vi "Begin.vi"(8 "error in":errorcluster) -> (0 "error out":errorcluster)   [LabVIEW 2023]
doc: "Called before other user functions, this VI can be used to open I/O refnums, load in file data, and do general program initialization. Notice that the <B>error out</B> terminal is simply used for data flow. Wiring it to other structures or subVIs ensures that this VI runs first."
uses:
  <vilib>/Rock Robotics/WPI/DriverStation/WPI_DriverStationRobotMode2.ctl
  <vilib>/Rock Robotics/WPI/Joystick/WPI_JoystickDeviceEnum.ctl
  Swerve/Implementation/Swerve Setpoints2.ctl
  Swerve/Implementation/Swerve Operations.ctl
  <vilib>/Rock Robotics/SystemInterfaces/DIO/FPGA_DIOChannel.ctl
  <vilib>/Rock Robotics/WPI/SafetyOutput/WPI_SafetyOutputConfigMenu.ctl
  <vilib>/Rock Robotics/WPI/ThirdParty/REV Robotics/REVLib/Typedef/Spark MAX Sensor Type.ctl
  <vilib>/Rock Robotics/WPI/ThirdParty/Phoenix-LabVIEW/Motor Controller/Controls/CTRE_Phoenix_MotorControl_NeutralMode.ctl
  <vilib>/Rock Robotics/WPI/ThirdParty/REV Robotics/REVLib/Typedef/Spark MAX Idle Mode.ctl
  Robot Global Data.vi
  <vilib>/Rock Robotics/Network Tables/NT Write String Array.vi
  <vilib>/Rock Robotics/SystemInterfaces/DIO/FPGA_DIOPWMChannel.ctl
panel:
  in  "Swerve PID":T1={"P Gain"=1.1, "I Gain"=0.0, "D Gain"=0.0, "F Gain"=0.0, "I Zone"=0.0, "Min Output"=-1.0, "Max Output"=1.0}
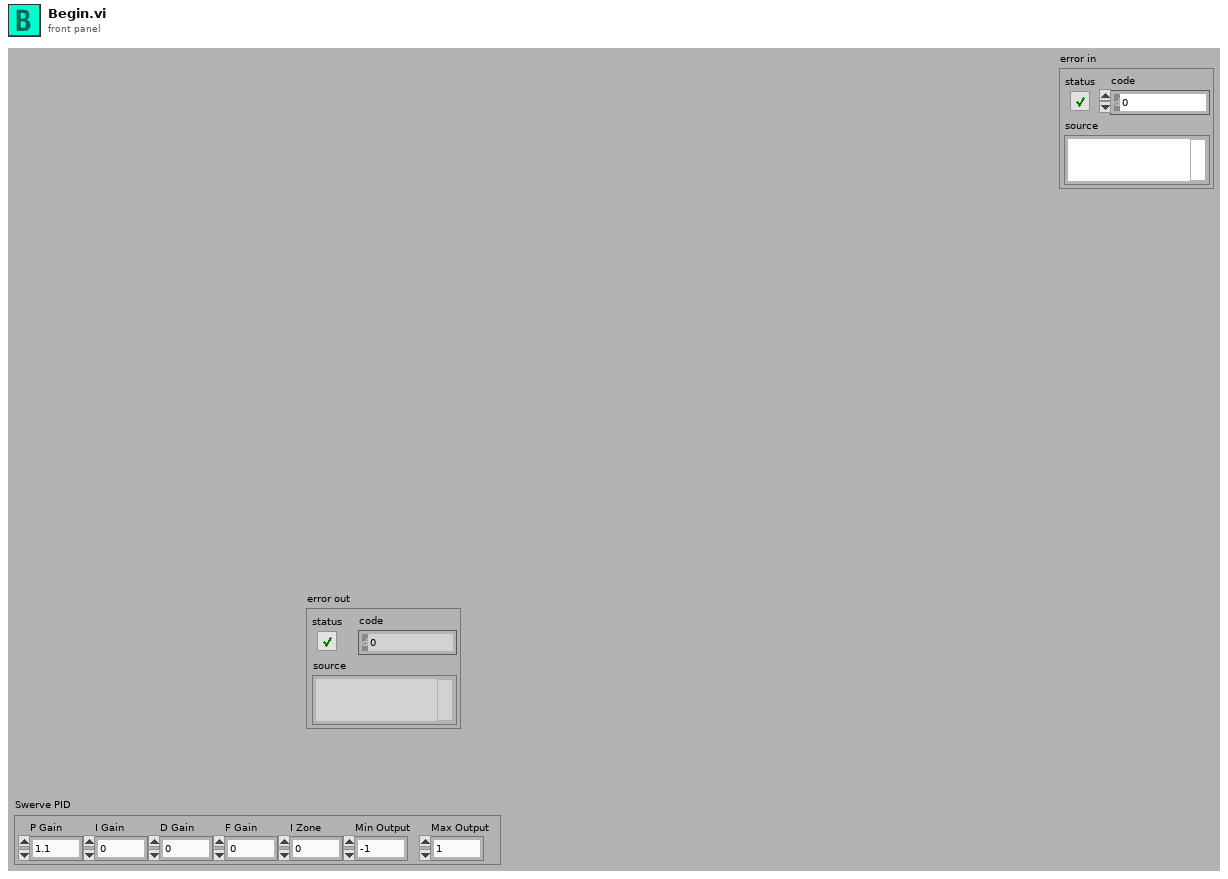
[diagram p1: front panel]
types:
  T1 = cluster{"P Gain":dbl, "I Gain":dbl, "D Gain":dbl, "F Gain":dbl, "I Zone":dbl, "Min Output":dbl, "Max Output":dbl}
  T2 = typedef "FPGA_DIOChannel.ctl" = enum8{"DIO 0", "DIO 1", "DIO 2", "DIO 3", "DIO 4", "DIO 5", "DIO 6", "DIO 7", "DIO 8", "DIO 9", "DIO MXP 0", "DIO MXP 1", "DIO MXP 2", "DIO MXP 3", "DIO MXP 4", "DIO MXP 5", "DIO MXP 6", "DIO MXP 7", "DIO MXP 8", "DIO MXP 9", "DIO MXP 10", "DIO MXP 11", "DIO MXP 12", "DIO MXP 13", "DIO MXP 14", "DIO MXP 15", "SPI Port CS1", "SPI Port CS2", "SPI Port CS3", "SPI Port MISO", "SPI Port MOSI", "Invalid"}
  T3 = typedef "Swerve Setpoints2.ctl" = cluster{"Operation":T4, "Gyro":dbl, "FWD":dbl, "STR":dbl, "X rotate":dbl, "Y rotate":dbl, "Time":dbl, "Distance":dbl, "Right Trigger":dbl, "Angle":dbl, "Start Angle":dbl, "Tag ID":dbl, "Start Positions":dbl[]}
  T4 = typedef "Swerve Operations.ctl" = enum16{"Reserve", "Read Current", "Immediate", "Stop", "Balance", "Direct  Joystick Drive", "Joystick Drive", "Drive for Distance", "Drive for Time", "Turn to Angle", "Drive to Angle(Time)", "Drive to Angle(Distance)", "Look At Cone", "Look At Cube", "Move To Tape", "Move To Tag"}
  T5 = typedef "WPI_JoystickDeviceEnum.ctl" = enum16{"USB 0", "USB 1", "USB 2", "USB 3", "USB 4", "USB 5"}
  T6 = typedef "WPI_DriverStationRobotMode2.ctl" = enum16{"Autonomous Disabled", "Autonomous Enabled", "Teleop Disabled", "Teleop Enabled", "Disconnected", "Finish", "Test Disabled", "Test Enabled", "Emergency Stopped"}
  T7 = typedef "Spark MAX Sensor Type.ctl" = enum16{"No Sensor", "Hall Sensor", "Encoder", "-Not Available-", "Analog", "Alternate Encoder", "Duty Cycle"}
  T8 = typedef "Spark MAX Idle Mode.ctl" = enum16{"Coast", "Brake"}
  T9 = typedef "WPI_SafetyOutputConfigMenu.ctl" = enum16{"Enable", "Disable"}
  T10 = typedef "WPI_MotorControlDeviceRef.ctl" = cluster{"DeviceStatus":errorcluster, "Type":T11, "PWM":cluster{"PWM Channel":T12, "DeadBand":T13}, "CAN":cluster{"Device Number":u8, "SetOutput VI Ref":variant, "GetOutput VI Ref":variant, "Enable VI Ref":variant, "Disable VI Ref":variant, "Data":variant}, "Invert":bool, "DIO PWM":cluster{"PWM \"Enable\" Channel":T12, "DIOChannel":T2, "PWM Rate":dbl}}
  T11 = typedef "WPI_MotorControlType.ctl" = enum16{"PWM", "CAN", "DIO PWM"}
  T12 = typedef "FPGA_DIOPWMChannel.ctl" = enum8{"PWM 0", "PWM 1", "PWM 2", "PWM 3", "PWM 4", "PWM 5", "PWM 6", "PWM 7", "PWM 8", "PWM 9", "PWM MXP 0", "PWM MXP 1", "PWM MXP 2", "PWM MXP 3", "PWM MXP 4", "PWM MXP 5", "PWM MXP 6", "PWM MXP 7", "PWM MXP 8", "PWM MXP 9", "Invalid"}
  T13 = typedef "WPI_PWMDeadband.ctl" = cluster{"Name":string, "maxPositivePwm":i32, "minPositivePwm":i32, "centerPwm":i32, "maxNegativePwm":i32, "minNegativePwm":i32, "angularRange":u16}
  T14 = typedef "WPI_JoystickDevRef.ctl" = cluster{"Device":T5}
  T15 = typedef "ADIS16470 Device Reference.ctl" = cluster{"DevStatus":errorcluster, "Hardware Config":T16, "Calibration Complete":refnum<notifier>, "Status Reference":refnum<data-value>, "Data Reference":refnum<data-value>, "Sychronous Process VI":T19, "Cmd FIFO":refnum<k33>, "Source":T20, "Data FIFO":refnum<k33>, "Calibration Time (ms)":u32, "Data Reference":refnum<data-value>}
  T16 = typedef "ADIS16470 Hardware Configuration.ctl" = cluster{"SPI Clock Rate (Hz)":dbl, "IMU SPI Mode (3)":T17, "IMU Reset Pin":T2, "IMU SPI Bus":T18, "IMU Data Ready Pin":T2, "Stall Config":cluster{"Pow2BytesPerRead":u8, "StallTicks":u16, "CsToSclkTicks":u8}}
  T17 = typedef "WPI_SPIMode.ctl" = enum16{"Mode 0 (Clk Idle Low,Sample on Leading)", "Mode 1 (Clk Idle Low,Sample on Trailing)", "Mode 2 (Clk Idle High,Sample on Leading)", "Mode 3 (Clk Idle High,Sample on Trailing)"}
  T18 = typedef "spi_bus.ctl" = enum16{"SPI On-Board, CS0", "SPI On-Board, CS1", "SPI On-Board, CS2", "SPI On-Board, CS3", "SPI MXP", "Invalid"}
  T19 = typedef "ADIS16470 Process.ctl" = refnum<vi>
  T20 = typedef "FPGA_CounterEncoderSourceConvertionLVSourceType.ctl" = cluster{"DevStatus":errorcluster, "AnalogTriggerMode?":bool, "DigitalMode":cluster{"DIO Channel":T21}, "AnalogTriggerMode":cluster{"AnalogTriggerIndex":T22, "OutputType":T23}}
  T21 = typedef "FPGA_DIODigitalSourceChannel.ctl" = enum8{"DIO 0", "DIO 1", "DIO 2", "DIO 3", "DIO 4", "DIO 5", "DIO 6", "DIO 7", "DIO 8", "DIO 9", "DIO MXP 0", "DIO MXP 1", "DIO MXP 2", "DIO MXP 3", "DIO MXP 4", "DIO MXP 5", "DIO MXP 6", "DIO MXP 7", "DIO MXP 8", "DIO MXP 9", "DIO MXP 10", "DIO MXP 11", "DIO MXP 12", "DIO MXP 13", "DIO MXP 14", "DIO MXP 15", "SPI Port CS1", "SPI Port CS2", "SPI Port CS3", "SPI Port MISO", "SPI Port MOSI", "Disabled"}
  T22 = typedef "FPGA_AnalogTriggerIndex.ctl" = enum8{"Trig 0", "Trig 1", "Trig 2", "Trig 3", "Trig 4", "Trig 5", "Trig 6", "Trig 7", "Invalid"}
  T23 = typedef "FPGA_AnalogTriggerOutType.ctl" = enum16{"InWindow", "TriggerState", "Rising", "Falling"}
  T24 = typedef "WPI_DigitalInputDevRef.ctl" = cluster{"DevStatus":errorcluster, "DIO Channel":T2}
  T25 = typedef "CTRE_Phoenix_MotorControl_NeutralMode.ctl" = enum8{"EEPROMSetting", "Override to Coast", "Override to Brake"}
  T26 = typedef "WPI_PWMDeviceRef.ctl" = cluster{"DeviceStatus":errorcluster, "PWM Channel":T12}
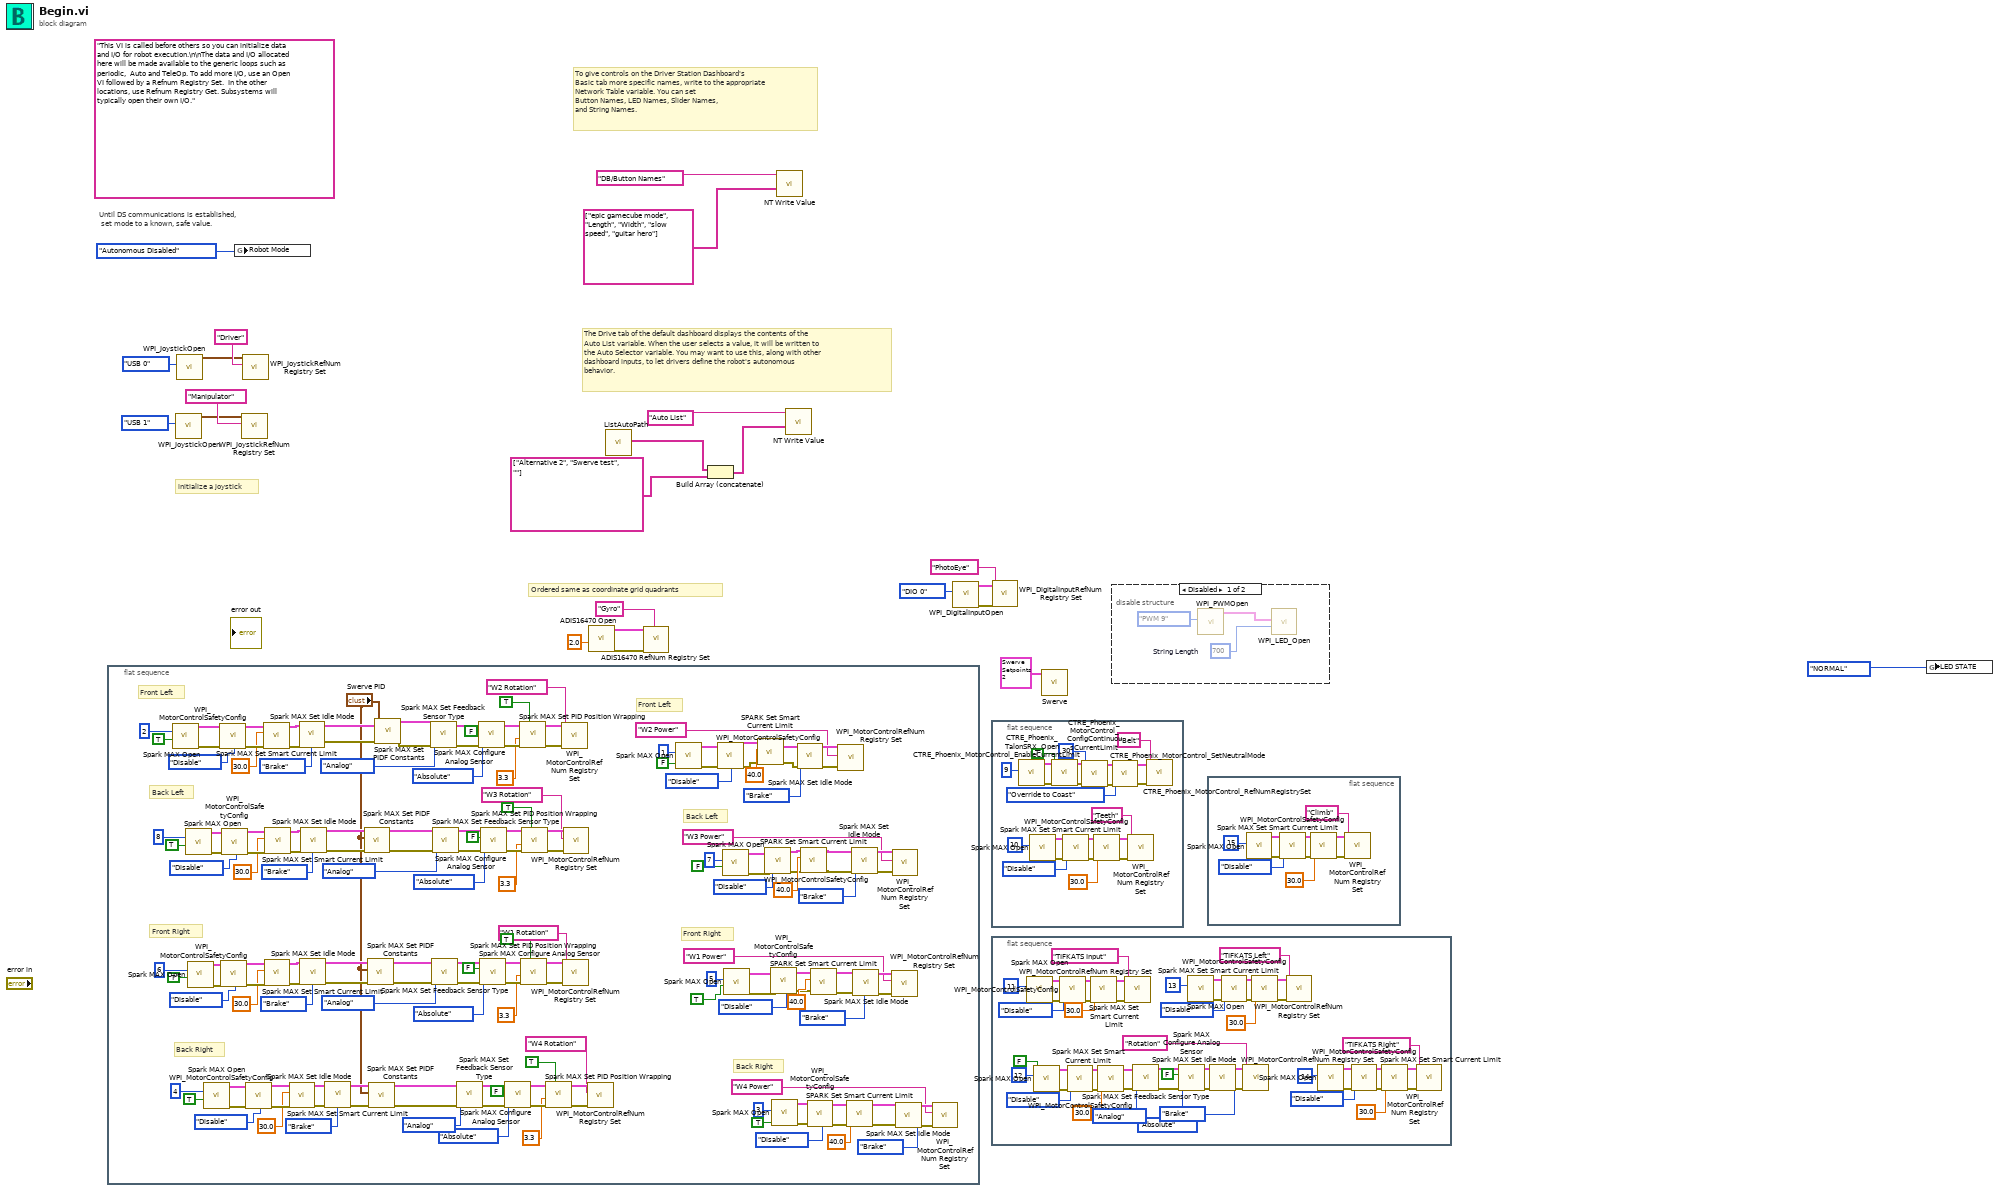
[diagram p0: block diagram]
diagram:
  (unwired) "This VI is called before others so you can initialize data and I/O for robot execution.\n\nThe data and I/O allocated here will be made available to the generic loops such as periodic,  Auto and TeleOp. To add more I/O, use an Open VI followed by a Refnum Registry Set.  In the other locations, use Refnum Registry Get. Subsystems will typically open their own I/O."
  # "Ordered same as coordinate grid quadrants"
  # "The Drive tab of the default dashboard displays the contents of the\nAuto List variable. When the user selects a value, it will be written to\nthe Auto Selector variable. You may want to use this, along with other\ndashboard inputs, to let drivers define the robot's autonomous\nbehavior."
  # "To give controls on the Driver Station Dashboard's\nBasic tab more specific names, write to the appropriate\nNetwork Table variable. You can set\nButton Names, LED Names, Slider Names,\nand String Names."
  # "initialize a joystick"
  # "Until DS communications is established,\n set mode to a known, safe value."
  n1 = flat-sequence {
    frame #0 {
      # "Back Right"
      # "Back Right"
      # "Front Right"
      # "Front Right"
      # "Back Left"
      # "Back Left"
      # "Front Left"
      # "Front Left"
      n2 = call <vilib>:"Spark MAX Open.vi"("Invert"=TRUE, "Device Number"=u8 2) -> ("error out"=w106:errorcluster, "MotorControlDeviceRef"=w107:T10)  [unwired: 8 in]
      n3 = call <vilib>:"Spark MAX Open.vi"("Invert"=TRUE, "Device Number"=u8 8) -> ("error out"=w170:errorcluster, "MotorControlDeviceRef"=w171:T10)  [unwired: 8 in]
      n4 = call <vilib>:"Spark MAX Open.vi"("Invert"=TRUE, "Device Number"=u8 6) -> ("error out"=w86:errorcluster, "MotorControlDeviceRef"=w87:T10)  [unwired: 8 in]
      n5 = call <vilib>:"Spark MAX Open.vi"("Invert"=TRUE, "Device Number"=u8 4) -> ("error out"=w66:errorcluster, "MotorControlDeviceRef"=w67:T10)  [unwired: 8 in]
      n6 = call <vilib>:"WPI_MotorControlSafetyConfig.vi"("error in (no error)"=w106, "mode"=WPI_SafetyOutputConfigMenu."Disable", "MotorControlDevRef"=w107) -> ("error out"=w124:errorcluster, "MotorControlDevRef"=w122:T10)  [unwired: 7 in]
      n7 = call <vilib>:"WPI_MotorControlSafetyConfig.vi"("error in (no error)"=w86, "mode"=WPI_SafetyOutputConfigMenu."Disable", "MotorControlDevRef"=w87) -> ("error out"=w104:errorcluster, "MotorControlDevRef"=w102:T10)  [unwired: 7 in]
      n8 = call <vilib>:"WPI_MotorControlSafetyConfig.vi"("error in (no error)"=w170, "mode"=WPI_SafetyOutputConfigMenu."Disable", "MotorControlDevRef"=w171) -> ("error out"=w178:errorcluster, "MotorControlDevRef"=w174:T10)  [unwired: 7 in]
      n9 = call <vilib>:"WPI_MotorControlSafetyConfig.vi"("error in (no error)"=w66, "mode"=WPI_SafetyOutputConfigMenu."Disable", "MotorControlDevRef"=w67) -> ("error out"=w84:errorcluster, "MotorControlDevRef"=w82:T10)  [unwired: 7 in]
      n10 = call <vilib>:"Spark MAX Set Smart Current Limit.vi"("error in (no error)"=w124, "Primay Current Limit (80A)"=30.0, "MotorControlDeviceRef in"=w122) -> ("error out"=w125:errorcluster, "MotorControlDeviceRef out"=w123:T10)  [unwired: 7 in]
      n11 = call <vilib>:"Spark MAX Set Smart Current Limit.vi"("error in (no error)"=w104, "Primay Current Limit (80A)"=30.0, "MotorControlDeviceRef in"=w102) -> ("error out"=w105:errorcluster, "MotorControlDeviceRef out"=w103:T10)  [unwired: 7 in]
      n12 = call <vilib>:"Spark MAX Set Smart Current Limit.vi"("error in (no error)"=w178, "Primay Current Limit (80A)"=30.0, "MotorControlDeviceRef in"=w174) -> ("error out"=w179:errorcluster, "MotorControlDeviceRef out"=w175:T10)  [unwired: 7 in]
      n13 = call <vilib>:"Spark MAX Set Smart Current Limit.vi"("error in (no error)"=w84, "Primay Current Limit (80A)"=30.0, "MotorControlDeviceRef in"=w82) -> ("error out"=w85:errorcluster, "MotorControlDeviceRef out"=w83:T10)  [unwired: 7 in]
      n14 = call <vilib>:"Spark MAX Set Idle Mode.vi"("error in (no error)"=w125, "Idle Mode"=Spark_MAX_Idle_Mode."Brake", "MotorControlDeviceRef in"=w123) -> ("error out"=w57:errorcluster, "MotorControlDeviceRef out"=w56:T10)  [unwired: 7 in]
      n15 = call <vilib>:"Spark MAX Set Idle Mode.vi"("error in (no error)"=w105, "Idle Mode"=Spark_MAX_Idle_Mode."Brake", "MotorControlDeviceRef in"=w103) -> ("error out"=w49:errorcluster, "MotorControlDeviceRef out"=w50:T10)  [unwired: 7 in]
      n16 = call <vilib>:"Spark MAX Set Idle Mode.vi"("error in (no error)"=w179, "Idle Mode"=Spark_MAX_Idle_Mode."Brake", "MotorControlDeviceRef in"=w175) -> ("error out"=w53:errorcluster, "MotorControlDeviceRef out"=w54:T10)  [unwired: 7 in]
      n17 = call <vilib>:"Spark MAX Set Idle Mode.vi"("error in (no error)"=w85, "Idle Mode"=Spark_MAX_Idle_Mode."Brake", "MotorControlDeviceRef in"=w83) -> ("error out"=w45:errorcluster, "MotorControlDeviceRef out"=w46:T10)  [unwired: 7 in]
      n18 = call <vilib>:"Spark MAX Set PIDF Constants.vi"("error in"=w53, "PID Constants"="Swerve PID", "MotorControlDeviceRef"=w54) -> ("error out"=w51:errorcluster, "MotorControlDeviceRef"=w52:T10)  [unwired: 7 in]
      n19 = call <vilib>:"Spark MAX Set PIDF Constants.vi"("error in"=w49, "PID Constants"="Swerve PID", "MotorControlDeviceRef"=w50) -> ("error out"=w47:errorcluster, "MotorControlDeviceRef"=w48:T10)  [unwired: 7 in]
      n20 = call <vilib>:"Spark MAX Set PIDF Constants.vi"("error in"=w45, "PID Constants"="Swerve PID", "MotorControlDeviceRef"=w46) -> ("error out"=w43:errorcluster, "MotorControlDeviceRef"=w44:T10)  [unwired: 7 in]
      n21 = call <vilib>:"Spark MAX Set PIDF Constants.vi"("error in"=w57, "PID Constants"="Swerve PID", "MotorControlDeviceRef"=w56) -> ("error out"=w58:errorcluster, "MotorControlDeviceRef"=w59:T10)  [unwired: 7 in]
      n22 = call <vilib>:"Spark MAX Set Feedback Sensor Type.vi"("error in (no error)"=w58, "Sensor Type"=Spark_MAX_Sensor_Type."Analog", "MotorControlDevRef"=w59) -> ("error out"=w115:errorcluster, "MotorControlDeviceRef"=w116:T10)  [unwired: 7 in]
      n23 = call <vilib>:"Spark MAX Set Feedback Sensor Type.vi"("error in (no error)"=w47, "Sensor Type"=Spark_MAX_Sensor_Type."Analog", "MotorControlDevRef"=w48) -> ("error out"=w95:errorcluster, "MotorControlDeviceRef"=w96:T10)  [unwired: 7 in]
      n24 = call <vilib>:"Spark MAX Set Feedback Sensor Type.vi"("error in (no error)"=w51, "Sensor Type"=Spark_MAX_Sensor_Type."Analog", "MotorControlDevRef"=w52) -> ("error out"=w134:errorcluster, "MotorControlDeviceRef"=w135:T10)  [unwired: 7 in]
      n25 = call <vilib>:"Spark MAX Set Feedback Sensor Type.vi"("error in (no error)"=w43, "Sensor Type"=Spark_MAX_Sensor_Type."Analog", "MotorControlDevRef"=w44) -> ("error out"=w75:errorcluster, "MotorControlDeviceRef"=w76:T10)  [unwired: 7 in]
      n26 = call <vilib>:"Spark MAX Configure Analog Sensor.vi"("error in (no error)"=w115, "Sensor Mode (Absolute)"=enum16{"Absolute", "Relative"}."Absolute", "Inverted (F)"=FALSE, "MotorControlDeviceRef in"=w116) -> ("error out"=w112:errorcluster, "MotorControlDeviceRef"=w113:T10)  [unwired: 6 in]
      n27 = call <vilib>:"Spark MAX Configure Analog Sensor.vi"("error in (no error)"=w95, "Sensor Mode (Absolute)"=enum16{"Absolute", "Relative"}."Absolute", "Inverted (F)"=FALSE, "MotorControlDeviceRef in"=w96) -> ("error out"=w92:errorcluster, "MotorControlDeviceRef"=w93:T10)  [unwired: 6 in]
      n28 = call <vilib>:"Spark MAX Configure Analog Sensor.vi"("error in (no error)"=w134, "Sensor Mode (Absolute)"=enum16{"Absolute", "Relative"}."Absolute", "Inverted (F)"=FALSE, "MotorControlDeviceRef in"=w135) -> ("error out"=w131:errorcluster, "MotorControlDeviceRef"=w132:T10)  [unwired: 6 in]
      n29 = call <vilib>:"Spark MAX Configure Analog Sensor.vi"("error in (no error)"=w75, "Sensor Mode (Absolute)"=enum16{"Absolute", "Relative"}."Absolute", "Inverted (F)"=FALSE, "MotorControlDeviceRef in"=w76) -> ("error out"=w72:errorcluster, "MotorControlDeviceRef"=w73:T10)  [unwired: 6 in]
      n30 = call <vilib>:"Spark MAX Set PID Position Wrapping.vi"("Enable (F)"=TRUE, "error in (no error)"=w112, "Maximum Output (0)"=3.3, "MotorControlDeviceRef in"=w113) -> ("error out"=w111:errorcluster, "MotorControlDeviceRef out"=w110:T10)  [unwired: 6 in]
      n31 = call <vilib>:"Spark MAX Set PID Position Wrapping.vi"("Enable (F)"=TRUE, "error in (no error)"=w92, "Maximum Output (0)"=3.3, "MotorControlDeviceRef in"=w93) -> ("error out"=w91:errorcluster, "MotorControlDeviceRef out"=w90:T10)  [unwired: 6 in]
      n32 = call <vilib>:"Spark MAX Set PID Position Wrapping.vi"("Enable (F)"=TRUE, "error in (no error)"=w131, "Maximum Output (0)"=3.3, "MotorControlDeviceRef in"=w132) -> ("error out"=w130:errorcluster, "MotorControlDeviceRef out"=w129:T10)  [unwired: 6 in]
      n33 = call <vilib>:"Spark MAX Set PID Position Wrapping.vi"("Enable (F)"=TRUE, "error in (no error)"=w72, "Maximum Output (0)"=3.3, "MotorControlDeviceRef in"=w73) -> ("error out"=w71:errorcluster, "MotorControlDeviceRef out"=w70:T10)  [unwired: 6 in]
      n34 = call <vilib>:"WPI_MotorControlRefNum Registry Set.vi"("error in (no error)"=w111, "refnum name"="W2 Rotation", "MotorControlDevRef"=w110) -> ()  [unwired: 7 in, 2 out]
      n35 = call <vilib>:"WPI_MotorControlRefNum Registry Set.vi"("error in (no error)"=w91, "refnum name"="W1 Rotation", "MotorControlDevRef"=w90) -> ()  [unwired: 7 in, 2 out]
      n36 = call <vilib>:"WPI_MotorControlRefNum Registry Set.vi"("error in (no error)"=w130, "refnum name"="W3 Rotation", "MotorControlDevRef"=w129) -> ()  [unwired: 7 in, 2 out]
      n37 = call <vilib>:"WPI_MotorControlRefNum Registry Set.vi"("error in (no error)"=w71, "refnum name"="W4 Rotation", "MotorControlDevRef"=w70) -> ()  [unwired: 7 in, 2 out]
      n38 = call <vilib>:"Spark MAX Open.vi"("Invert"=FALSE, "Device Number"=u8 1) -> ("error out"=w185:errorcluster, "MotorControlDeviceRef"=w186:T10)  [unwired: 8 in]
      n39 = call <vilib>:"WPI_MotorControlSafetyConfig.vi"("error in (no error)"=w185, "mode"=WPI_SafetyOutputConfigMenu."Disable", "MotorControlDevRef"=w186) -> ("error out"=w24:errorcluster, "MotorControlDevRef"=w34:T10)  [unwired: 7 in]
      n40 = call <vilib>:"Spark MAX Open.vi"("Invert"=FALSE, "Device Number"=u8 7) -> ("error out"=w172:errorcluster, "MotorControlDeviceRef"=w173:T10)  [unwired: 8 in]
      n41 = call <vilib>:"Spark MAX Open.vi"("Invert"=TRUE, "Device Number"=u8 5) -> ("error out"=w158:errorcluster, "MotorControlDeviceRef"=w159:T10)  [unwired: 8 in]
      n42 = call <vilib>:"SPARK Set Smart Current Limit.vi"("error in (no error)"=w24, "Primay Current Limit (80A)"=40.0, "MotorControlDeviceRef in"=w34) -> ("error out"=w32:errorcluster, "MotorControlDeviceRef out"=w35:T10)  [unwired: 7 in]
      n43 = call <vilib>:"WPI_MotorControlSafetyConfig.vi"("error in (no error)"=w172, "mode"=WPI_SafetyOutputConfigMenu."Disable", "MotorControlDevRef"=w173) -> ("error out"=w25:errorcluster, "MotorControlDevRef"=w31:T10)  [unwired: 7 in]
      n44 = call <vilib>:"WPI_MotorControlSafetyConfig.vi"("error in (no error)"=w158, "mode"=WPI_SafetyOutputConfigMenu."Disable", "MotorControlDevRef"=w159) -> ("error out"=w27:errorcluster, "MotorControlDevRef"=w37:T10)  [unwired: 7 in]
      n45 = call <vilib>:"Spark MAX Open.vi"("Invert"=TRUE, "Device Number"=u8 3) -> ("error out"=w144:errorcluster, "MotorControlDeviceRef"=w145:T10)  [unwired: 8 in]
      n46 = call <vilib>:"Spark MAX Set Idle Mode.vi"("error in (no error)"=w32, "Idle Mode"=Spark_MAX_Idle_Mode."Brake", "MotorControlDeviceRef in"=w35) -> ("error out"=w187:errorcluster, "MotorControlDeviceRef out"=w188:T10)  [unwired: 7 in]
      n47 = call <vilib>:"SPARK Set Smart Current Limit.vi"("error in (no error)"=w25, "Primay Current Limit (80A)"=40.0, "MotorControlDeviceRef in"=w31) -> ("error out"=w28:errorcluster, "MotorControlDeviceRef out"=w29:T10)  [unwired: 7 in]
      n48 = call <vilib>:"WPI_MotorControlSafetyConfig.vi"("error in (no error)"=w144, "mode"=WPI_SafetyOutputConfigMenu."Disable", "MotorControlDevRef"=w145) -> ("error out"=w146:errorcluster, "MotorControlDevRef"=w147:T10)  [unwired: 7 in]
      n49 = call <vilib>:"SPARK Set Smart Current Limit.vi"("error in (no error)"=w27, "Primay Current Limit (80A)"=40.0, "MotorControlDeviceRef in"=w37) -> ("error out"=w26:errorcluster, "MotorControlDeviceRef out"=w38:T10)  [unwired: 7 in]
      n50 = call <vilib>:"WPI_MotorControlRefNum Registry Set.vi"("error in (no error)"=w187, "refnum name"="W2 Power", "MotorControlDevRef"=w188) -> ()  [unwired: 7 in, 2 out]
      n51 = call <vilib>:"SPARK Set Smart Current Limit.vi"("error in (no error)"=w146, "Primay Current Limit (80A)"=40.0, "MotorControlDeviceRef in"=w147) -> ("error out"=w148:errorcluster, "MotorControlDeviceRef out"=w149:T10)  [unwired: 7 in]
      n52 = call <vilib>:"Spark MAX Set Idle Mode.vi"("error in (no error)"=w28, "Idle Mode"=Spark_MAX_Idle_Mode."Brake", "MotorControlDeviceRef in"=w29) -> ("error out"=w177:errorcluster, "MotorControlDeviceRef out"=w176:T10)  [unwired: 7 in]
      n53 = call <vilib>:"Spark MAX Set Idle Mode.vi"("error in (no error)"=w26, "Idle Mode"=Spark_MAX_Idle_Mode."Brake", "MotorControlDeviceRef in"=w38) -> ("error out"=w160:errorcluster, "MotorControlDeviceRef out"=w161:T10)  [unwired: 7 in]
      n54 = call <vilib>:"WPI_MotorControlRefNum Registry Set.vi"("error in (no error)"=w160, "refnum name"="W1 Power", "MotorControlDevRef"=w161) -> ()  [unwired: 7 in, 2 out]
      n55 = call <vilib>:"WPI_MotorControlRefNum Registry Set.vi"("error in (no error)"=w177, "refnum name"="W3 Power", "MotorControlDevRef"=w176) -> ()  [unwired: 7 in, 2 out]
      n56 = call <vilib>:"Spark MAX Set Idle Mode.vi"("error in (no error)"=w148, "Idle Mode"=Spark_MAX_Idle_Mode."Brake", "MotorControlDeviceRef in"=w149) -> ("error out"=w150:errorcluster, "MotorControlDeviceRef out"=w151:T10)  [unwired: 7 in]
      n57 = call <vilib>:"WPI_MotorControlRefNum Registry Set.vi"("error in (no error)"=w150, "refnum name"="W4 Power", "MotorControlDevRef"=w151) -> ()  [unwired: 7 in, 2 out]
    }
  }
  n58 = call <vilib>:"WPI_JoystickOpen.vi"("JoystickDevice"=WPI_JoystickDeviceEnum."USB 1") -> ("JoystickDevRef"=w15:T14)  [unwired: 10 in]
  n59 = call <vilib>:"WPI_JoystickOpen.vi"("JoystickDevice"=WPI_JoystickDeviceEnum."USB 0") -> ("JoystickDevRef"=w21:T14)  [unwired: 10 in]
  n60 = global write "Robot Global Data.vi" "Robot Mode"(WPI_DriverStationRobotMode2."Autonomous Disabled" ("Robot Mode")) -> ()
  n61 = call <vilib>:"WPI_JoystickRefNum Registry Set.vi"("refnum name"="Manipulator", "JoystickDevRef"=w15) -> ()  [unwired: 8 in, 2 out]
  n62 = call <vilib>:"WPI_JoystickRefNum Registry Set.vi"("refnum name"="Driver", "JoystickDevRef"=w21) -> ()  [unwired: 8 in, 2 out]
  n63 = call <vilib>:"ADIS16470 Open.vi"("Initial Calibration Time (4s)"=2.0) -> ("error out"=w2:errorcluster, "ADIS16470DevRef"=w10:T15)  [unwired: 9 in]
  n64 = call "ListAutoPath.vi"() -> ("AutoRoutinesNames"=w12:string[])  [unwired: 11 in]
  n65 = call <vilib>:"ADIS16470 RefNum Registry Set.vi"("error in (no error)"=w2, "refnum name"="Gyro", "ADIS16470DevRef in"=w10) -> ()  [unwired: 7 in, 2 out]
  n66 = Build Array (concatenate)(w12, string[] ["Alternative 2", "Swerve test", ""] ("String Array")) -> (w13:string[])
  n67 = call-poly <vilib>:"NT Write Value.vi"("value"=string[] ["epic gamecube mode", "Length", "Width", "slow speed", "guitar hero"] ("String Array"), "name"="DB/Button Names" ("Name")) -> ()  [unwired: 9 in, 1 out]
  n68 = call-poly <vilib>:"NT Write Value.vi"("value"=w13, "name"="Auto List" ("Name")) -> ()  [unwired: 9 in, 1 out]
  n69 = call <vilib>:"WPI_DigitalInputOpen.vi"("DIO Channel"=FPGA_DIOChannel."DIO 0") -> ("error out"=w6:errorcluster, "DigitalInputDevRef"=w5:T24)  [unwired: 9 in]
  n70 = flat-sequence {
    frame #0 {
      n71 = call <vilib>:"CTRE_Phoenix_TalonSRX_Open.vi"("Device Number"=u8 9) -> ("error out"=w199:errorcluster, "PhoenixMotorControlDevRef"=w198:T10)  [unwired: 9 in]
      n72 = call <vilib>:"Spark MAX Open.vi"("Device Number"=u8 10) -> ("error out"=w208:errorcluster, "MotorControlDeviceRef"=w209:T10)  [unwired: 9 in]
      n73 = call <vilib>:"CTRE_Phoenix_MotorControl_EnableCurrentLimit.vi"("error in (no error)"=w199, "Enable Current Limit?"=TRUE, "PhoenixMotorControlDevRef"=w198) -> ("error out"=w197:errorcluster, "PhoenixMotorControlDevRef"=w196:T10)  [unwired: 7 in]
      n74 = call <vilib>:"WPI_MotorControlSafetyConfig.vi"("error in (no error)"=w208, "mode"=WPI_SafetyOutputConfigMenu."Disable", "MotorControlDevRef"=w209) -> ("error out"=w205:errorcluster, "MotorControlDevRef"=w206:T10)  [unwired: 7 in]
      n75 = call <vilib>:"CTRE_Phoenix_MotorControl_ConfigContinuousCurrentLimit.vi"("error in (no error)"=w197, "Continuous Current Limit (Amps)"=30, "PhoenixMotorControlDevRef"=w196) -> ("error out"=w194:errorcluster, "PhoenixMotorControlDevRef"=w193:T10)  [unwired: 7 in]
      n76 = call <vilib>:"Spark MAX Set Smart Current Limit.vi"("error in (no error)"=w205, "Primay Current Limit (80A)"=30.0, "MotorControlDeviceRef in"=w206) -> ("error out"=w203:errorcluster, "MotorControlDeviceRef out"=w204:T10)  [unwired: 7 in]
      n77 = call <vilib>:"CTRE_Phoenix_MotorControl_SetNeutralMode.vi"("error in (no error)"=w194, "Motor Control Neutral Mode"=CTRE_Phoenix_MotorControl_NeutralMode."Override to Coast", "PhoenixMotorControlDevRef"=w193) -> ("error out"=w191:errorcluster, "PhoenixMotorControlDevRef"=w192:T10)  [unwired: 7 in]
      n78 = call <vilib>:"WPI_MotorControlRefNum Registry Set.vi"("error in (no error)"=w203, "refnum name"="Teeth", "MotorControlDevRef"=w204) -> ()  [unwired: 7 in, 2 out]
      n79 = call <vilib>:"CTRE_Phoenix_MotorControl_RefNumRegistrySet.vi"("error in (no error)"=w191, "refnum name"="Belt", "PhoenixMotorControlDevRef"=w192) -> ()  [unwired: 7 in, 2 out]
    }
  }
  n80 = flat-sequence {
    frame #0 {
      n81 = call <vilib>:"Spark MAX Open.vi"("Device Number"=u8 11) -> ("error out"=w261:errorcluster, "MotorControlDeviceRef"=w262:T10)  [unwired: 9 in]
      n82 = call <vilib>:"Spark MAX Open.vi"("Invert"=FALSE, "Device Number"=u8 12) -> ("error out"=w231:errorcluster, "MotorControlDeviceRef"=w232:T10)  [unwired: 8 in]
      n83 = call <vilib>:"WPI_MotorControlSafetyConfig.vi"("error in (no error)"=w261, "mode"=WPI_SafetyOutputConfigMenu."Disable", "MotorControlDevRef"=w262) -> ("error out"=w258:errorcluster, "MotorControlDevRef"=w259:T10)  [unwired: 7 in]
      n84 = call <vilib>:"WPI_MotorControlSafetyConfig.vi"("error in (no error)"=w231, "mode"=WPI_SafetyOutputConfigMenu."Disable", "MotorControlDevRef"=w232) -> ("error out"=w228:errorcluster, "MotorControlDevRef"=w229:T10)  [unwired: 7 in]
      n85 = call <vilib>:"Spark MAX Set Smart Current Limit.vi"("error in (no error)"=w258, "Primay Current Limit (80A)"=30.0, "MotorControlDeviceRef in"=w259) -> ("error out"=w256:errorcluster, "MotorControlDeviceRef out"=w257:T10)  [unwired: 7 in]
      n86 = call <vilib>:"Spark MAX Set Smart Current Limit.vi"("error in (no error)"=w228, "Primay Current Limit (80A)"=30.0, "MotorControlDeviceRef in"=w229) -> ("error out"=w219:errorcluster, "MotorControlDeviceRef out"=w218:T10)  [unwired: 7 in]
      n87 = call <vilib>:"WPI_MotorControlRefNum Registry Set.vi"("error in (no error)"=w256, "refnum name"="TIFKATS Input", "MotorControlDevRef"=w257) -> ()  [unwired: 7 in, 2 out]
      n88 = call <vilib>:"Spark MAX Set Feedback Sensor Type.vi"("error in (no error)"=w219, "Sensor Type"=Spark_MAX_Sensor_Type."Analog", "MotorControlDevRef"=w218) -> ("error out"=w221:errorcluster, "MotorControlDeviceRef"=w222:T10)  [unwired: 7 in]
      n89 = call <vilib>:"Spark MAX Configure Analog Sensor.vi"("error in (no error)"=w221, "Sensor Mode (Absolute)"=enum16{"Absolute", "Relative"}."Absolute", "Inverted (F)"=FALSE, "MotorControlDeviceRef in"=w222) -> ("error out"=w213:errorcluster, "MotorControlDeviceRef"=w214:T10)  [unwired: 6 in]
      n90 = call <vilib>:"Spark MAX Open.vi"("Device Number"=u8 13) -> ("error out"=w252:errorcluster, "MotorControlDeviceRef"=w253:T10)  [unwired: 9 in]
      n91 = call <vilib>:"Spark MAX Set Idle Mode.vi"("error in (no error)"=w213, "Idle Mode"=Spark_MAX_Idle_Mode."Brake", "MotorControlDeviceRef in"=w214) -> ("error out"=w212:errorcluster, "MotorControlDeviceRef out"=w215:T10)  [unwired: 7 in]
      n92 = call <vilib>:"WPI_MotorControlSafetyConfig.vi"("error in (no error)"=w252, "mode"=WPI_SafetyOutputConfigMenu."Disable", "MotorControlDevRef"=w253) -> ("error out"=w249:errorcluster, "MotorControlDevRef"=w250:T10)  [unwired: 7 in]
      n93 = call <vilib>:"WPI_MotorControlRefNum Registry Set.vi"("error in (no error)"=w212, "refnum name"="Rotation", "MotorControlDevRef"=w215) -> ()  [unwired: 7 in, 2 out]
      n94 = call <vilib>:"Spark MAX Set Smart Current Limit.vi"("error in (no error)"=w249, "Primay Current Limit (80A)"=30.0, "MotorControlDeviceRef in"=w250) -> ("error out"=w247:errorcluster, "MotorControlDeviceRef out"=w248:T10)  [unwired: 7 in]
      n95 = call <vilib>:"WPI_MotorControlRefNum Registry Set.vi"("error in (no error)"=w247, "refnum name"="TIFKATS Left", "MotorControlDevRef"=w248) -> ()  [unwired: 7 in, 2 out]
      n96 = call <vilib>:"Spark MAX Open.vi"("Device Number"=u8 14) -> ("error out"=w241:errorcluster, "MotorControlDeviceRef"=w242:T10)  [unwired: 9 in]
      n97 = call <vilib>:"WPI_MotorControlSafetyConfig.vi"("error in (no error)"=w241, "mode"=WPI_SafetyOutputConfigMenu."Disable", "MotorControlDevRef"=w242) -> ("error out"=w238:errorcluster, "MotorControlDevRef"=w239:T10)  [unwired: 7 in]
      n98 = call <vilib>:"Spark MAX Set Smart Current Limit.vi"("error in (no error)"=w238, "Primay Current Limit (80A)"=30.0, "MotorControlDeviceRef in"=w239) -> ("error out"=w236:errorcluster, "MotorControlDeviceRef out"=w237:T10)  [unwired: 7 in]
      n99 = call <vilib>:"WPI_MotorControlRefNum Registry Set.vi"("error in (no error)"=w236, "refnum name"="TIFKATS Right", "MotorControlDevRef"=w237) -> ()  [unwired: 7 in, 2 out]
    }
  }
  n100 = call <vilib>:"WPI_DigitalInputRefNum Registry Set.vi"("error in (no error)"=w6, "refnum name"="PhotoEye", "DigitalInputDevRef"=w5) -> ()  [unwired: 7 in, 2 out]
  n101 = call "Swerve.vi"("SubSystem Data"=T3 {"Operation"=enum."Joystick Drive", "Gyro"=0.0, "FWD"=0.0, "STR"=0.0, "X rotate"=0.0, "Y rotate"=0.0, "Time"=0.0, "Distance"=0.0, "Right Trigger"=0.0, "Angle"=0.0, "Start Angle"=0.0, "Tag ID"=0.0, "Start Positions"=[]}) -> ()  [unwired: 10 in, 1 out]
  n102 = disable-structure shown="Disabled" {
    frame Disabled {
      w263 = u16 700  # String Length
      n103 = call <vilib>:"WPI_PWMOpen.vi"("PWM Channel"=FPGA_DIOPWMChannel."PWM 9") -> ("PWMDeviceRef"=w265:T26)  [unwired: 9 in, 1 out]
      n104 = call <vilib>:"WPI_LED_Open.vi"("String Length"=w263, "PWMDeviceRef"=w265) -> ()  [unwired: 9 in, 1 out]
    }
    frame Enabled {
    }
  }
  n105 = flat-sequence {
    frame #0 {
      n106 = call <vilib>:"Spark MAX Open.vi"("Device Number"=u8 15) -> ("error out"=w274:errorcluster, "MotorControlDeviceRef"=w275:T10)  [unwired: 9 in]
      n107 = call <vilib>:"WPI_MotorControlSafetyConfig.vi"("error in (no error)"=w274, "mode"=WPI_SafetyOutputConfigMenu."Disable", "MotorControlDevRef"=w275) -> ("error out"=w271:errorcluster, "MotorControlDevRef"=w272:T10)  [unwired: 7 in]
      n108 = call <vilib>:"Spark MAX Set Smart Current Limit.vi"("error in (no error)"=w271, "Primay Current Limit (80A)"=30.0, "MotorControlDeviceRef in"=w272) -> ("error out"=w269:errorcluster, "MotorControlDeviceRef out"=w270:T10)  [unwired: 7 in]
      n109 = call <vilib>:"WPI_MotorControlRefNum Registry Set.vi"("error in (no error)"=w269, "refnum name"="Climb", "MotorControlDevRef"=w270) -> ()  [unwired: 7 in, 2 out]
    }
  }
  n110 = global write "Robot Global Data.vi" "LED STATE"(enum16{"NORMAL", "RAINBOW"}."NORMAL" ("LED STATE")) -> ()
